vi "Prueba Auto-Cycle.vi"() -> ()   [LabVIEW 2014, in "AD4212C.lvlib"]
uses:
  DriverMasterAsync/builds/DriverMasterAsync.lvlibp/APIs/Data Queue/Async Acquisition Data Cluster.ctl
  AD4212CClass/AD4212C.lvclass
  AD4212C.lvlib
  DriverMasterAsync/builds/DriverMasterAsync.lvlibp/Modules/HAL/DriverMasterAsync/DriverMasterAsyncClass/DriverMasterAsync.lvclass
  DriverMasterAsync/builds/DriverMasterAsync.lvlibp/APIs/Data Queue/WINFAS 2 Data Queue.lvlib
panel:
  out "error out":errorcluster
  out "ACQ Data":T1
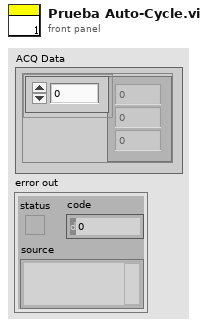
[diagram p1: front panel]
types:
  T1 = typedef "DriverMasterAsync.lvlibp/WINFAS 2 Data Queue.lvlib/Async Acquisition Data Cluster.ctl" = cluster{"Data":sgl[]}
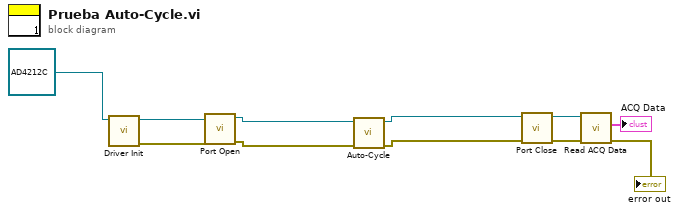
[diagram p0: block diagram]
diagram:
  n1 = call-dynamic "Driver Init.vi"("AD4212C in"=refnum<class "AD4212C.lvclass"> refnum ("AD4212C.lvlib:AD4212C.lvclass")) -> ("error out"=w5:errorcluster, "AD4212C out"=w7:refnum<class "AD4212C.lvclass">)  [unwired: 9 in]
  n2 = call-dynamic "Port Open.vi"("error in (no error)"=w5, "AD4212C in"=w7) -> ("error out"=w10:errorcluster, "AD4212C out"=w11:refnum<class "AD4212C.lvclass">)  [unwired: 8 in]
  n3 = call-dynamic "Auto-Cycle.vi"("error in (no error)"=w10, "AD4212C in"=w11) -> ("error out"=w9:errorcluster, "AD4212C out"=w8:refnum<class "AD4212C.lvclass">)  [unwired: 8 in]
  n4 = call-dynamic "Port Close.vi"("error in (no error)"=w9, "AD4212C in"=w8) -> ("error out"=w4:errorcluster, "AD4212C out"=w3:refnum<class "AD4212C.lvclass">)  [unwired: 8 in]
  n5 = call "Read ACQ Data.vi"("error in (no error)"=w4, "DriverMasterAsync in"=w3) -> ("error out"=→"error out":errorcluster, "ACQ Data"=→"ACQ Data":T1)  [unwired: 7 in, 1 out]
